vi "Load Related Entities.vi"(6 "Entity Manager in":refnum<class "Entity Manager.lvclass">, 11 "Entity Collection in":refnum<class "Entity Collection.lvclass">) -> (0 "error out":errorcluster, 3 "Entity Collection out":refnum<class "Entity Collection.lvclass">, 4 "Entity Manager":refnum<class "Entity Manager.lvclass">)   [LabVIEW 2020, in "Conditu2.lvlib" / "Columns.lvlib" / "Entity Collection.lvclass"]
uses:
  Entity Collection.lvclass
  C:/dev/lv20CE/lv-conditum-tools/Conditum-Clone/Columns/Relation/Relation.lvclass
  Entity Manager/Entity Manager.lvclass
  Relation/Relation.lvclass/Relation.ctl
  Entity Collection.lvclass/Entity Collection.ctl
  Entity ID.ctl
  Entity/Entity.lvclass/Entity.ctl
  ID/ID.lvclass/ID.ctl
  ID/Get.vi
  Relation/Relation.lvclass
  Conditu2.lvlib
  Entity/Entity.lvclass
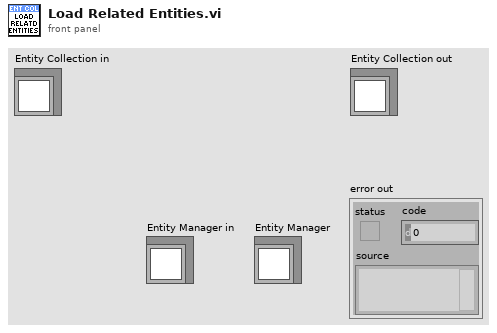
[diagram p1: front panel]
types:
  T1 = typedef "Conditu2.lvlib/Entity ID.ctl" = i64
  T2 = typedef "Conditu2.lvlib/Relation Info.ctl" = cluster{"Mapping":T3, "Related To":string, "Reversed By":string}
  T3 = typedef "Conditu2.lvlib/Relation Mapping.ctl" = enum16{"OneToOne", "OneToMany", "ManyToOne", "ManyToMany"}
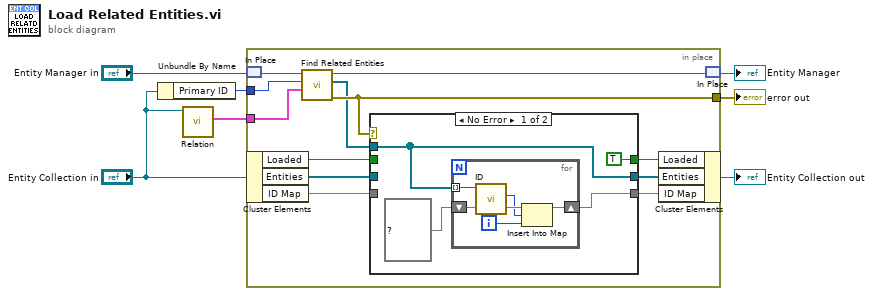
[diagram p0: block diagram]
diagram:
  n1 = Unbundle By Name("Entity Collection in") -> ("Primary ID"=w6:T1)
  n2 = call "Relation.vi"("Relation in"="Entity Collection in") -> ("Relation"=w1:T2)  [unwired: 10 in]
  n3 = in-place {
    in-place-border: w6 -> [w17]
    in-place-border: [w13] -> w5
    in-place-border: w1 -> [w16]
    n4 = in-place-match #1("Entity Manager in") -> (w19:refnum<class "Entity Manager.lvclass">)
    n5 = in-place-cluster #2("Entity Collection in") -> ("Loaded"=w15:bool, "Entities"=w14:refnum<class "Entity.lvclass">[], "ID Map"=w11:map{T1, i32})
    n6 = call "Find Related Entities.vi"("Relation"=w16, "Primary ID"=w17, "Entity Manager in"=w19) -> ("error out"=w13:errorcluster, "Entities"=w12:refnum<class "Entity.lvclass">[], "Entity Manager out"=w18:refnum<class "Entity Manager.lvclass">)  [unwired: 6 in]
    n7 = case shown="No Error" w13 {
      tunnel: w15 -> [_ w31]
      tunnel: w14 -> [_ w30]
      tunnel: w12 -> [w21 _]
      tunnel: w11 -> [_ w29]
      tunnel: [TRUE ("Loaded") w31] -> w10
      tunnel: [w21 w30] -> w9
      tunnel: [w20 w29] -> w8
      frame No Error {
        n8 = for {
          shift-right: [w24] -> w20
          shift-left: map{T1, i32} {} ("ID Map") -> [w27]
          tunnel: w21 -> [w28] mode=indexing
          i -> [w25]
          n9 = call "ID.vi"("Entity in"=w28) -> ("ID"=w26:T1)  [unwired: 9 in, 1 out]
          n10 = Insert Into Map(map in=w27, key=w26, value=w25) -> (map out=w24:map{T1, i32})  [unwired: 2 out]
        }
      }
      frame Error {
      }
    }
    n11 = in-place-cluster #2("Loaded"=w10, "Entities"=w9, "ID Map"=w8) -> (→"Entity Collection out":refnum<class "Entity Collection.lvclass">)
    n12 = in-place-match #1(w18) -> (→"Entity Manager":refnum<class "Entity Manager.lvclass">)
  }
  "error out" <- w5
